vi "AUTON_Index.vi"(0 "Auton Array":dbl[][](array[numeric]), 5 "MeasuredHeading":dbl, 7 "LeftEncoder":dbl, 9 "RightEncoder":dbl) -> (4 "Right Drive":dbl, 6 "Left Drive":dbl, 8 "Harvester":dbl, 10 "Winch":dbl, 14 "Roller":dbl, 15 "Cam":dbl)   [LabVIEW 2013]
uses:
  Robot Global Data.vi
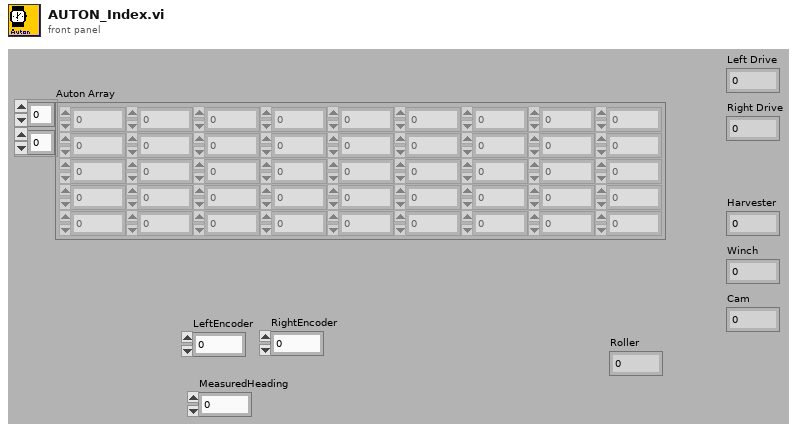
[diagram p1: front panel]
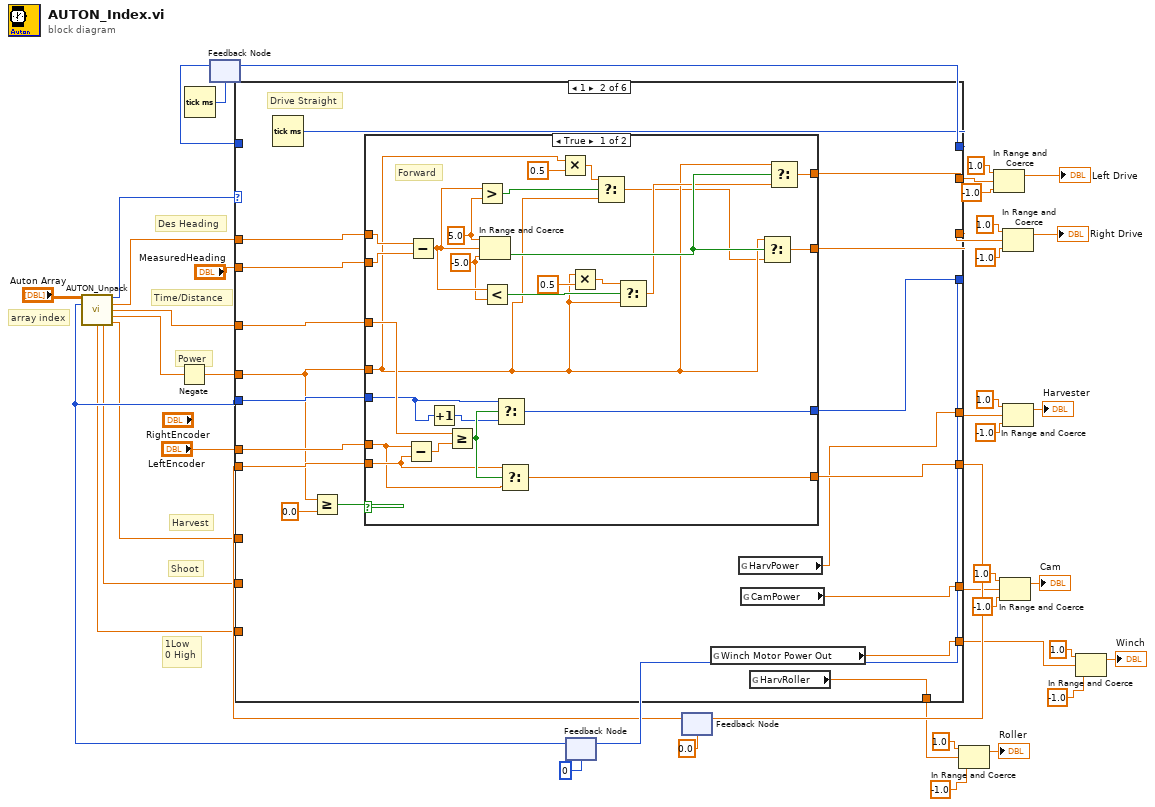
[diagram p0: block diagram]
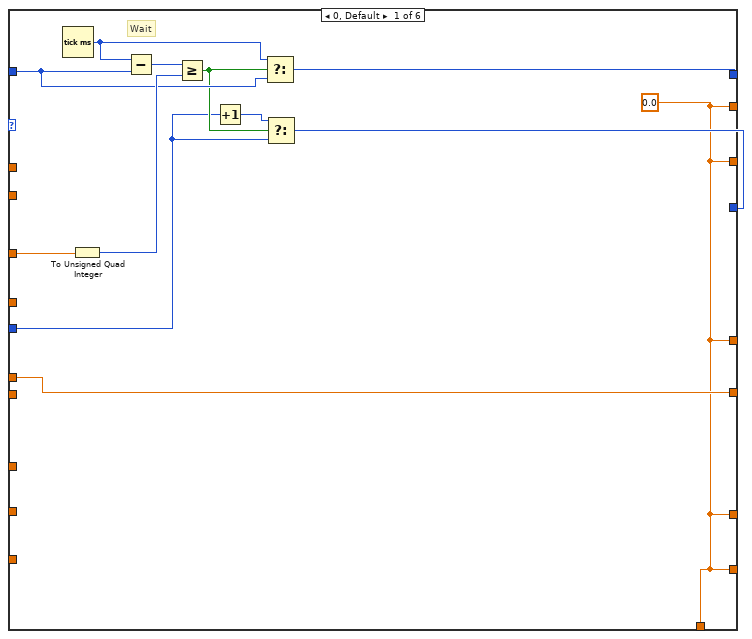
[diagram p2: hidden frame]
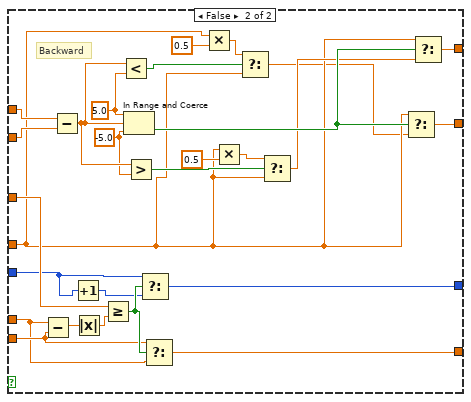
[diagram p3: hidden frame]
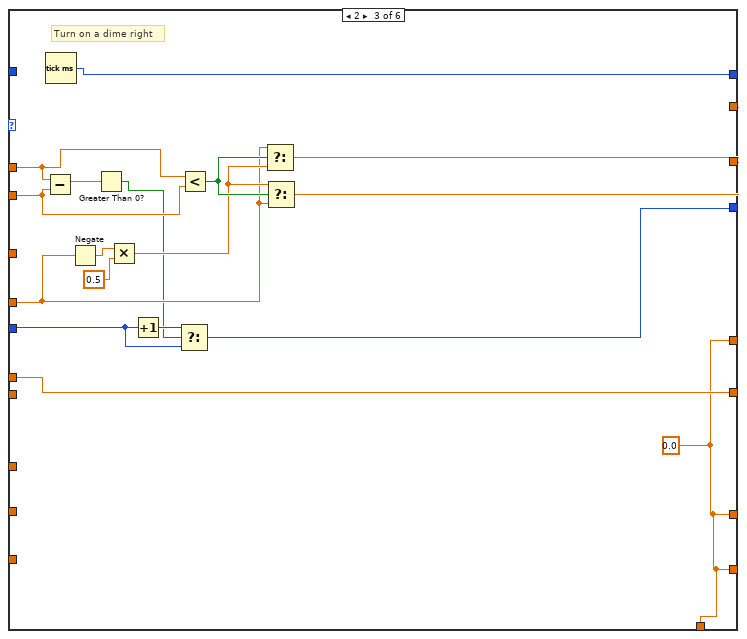
[diagram p4: hidden frame]
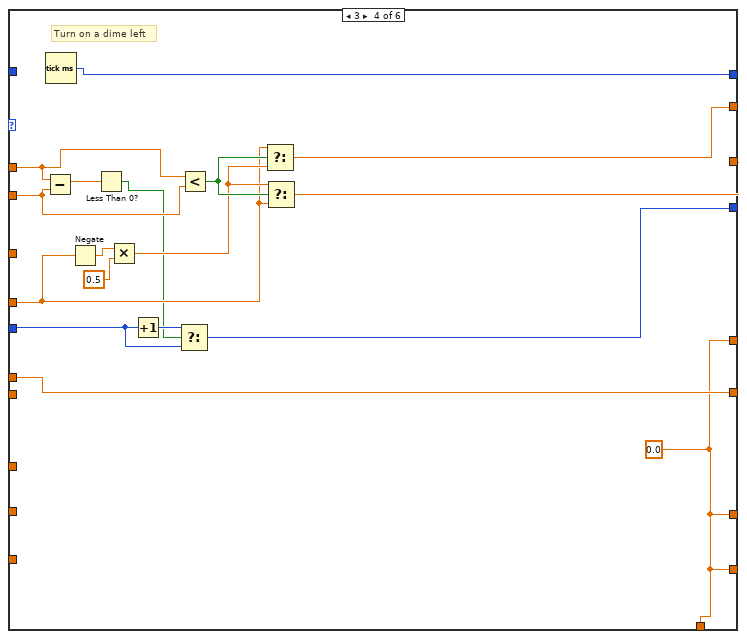
[diagram p5: hidden frame]
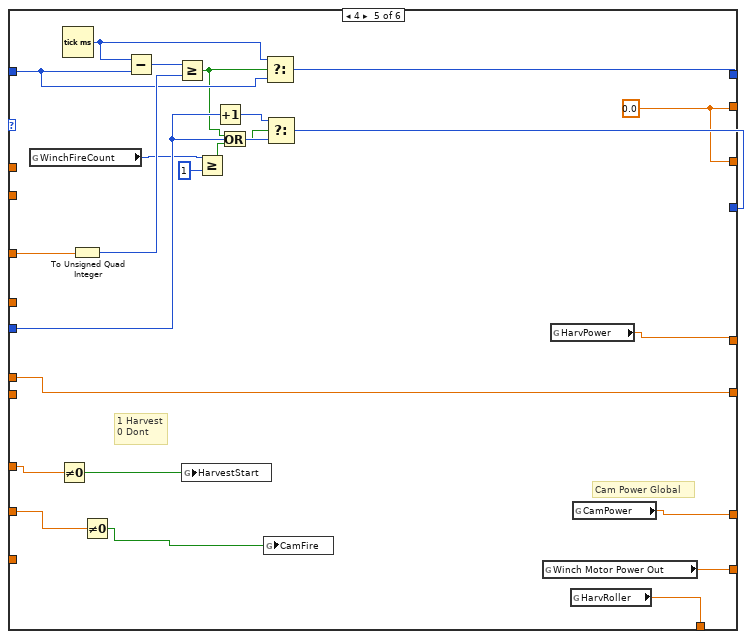
[diagram p6: hidden frame]
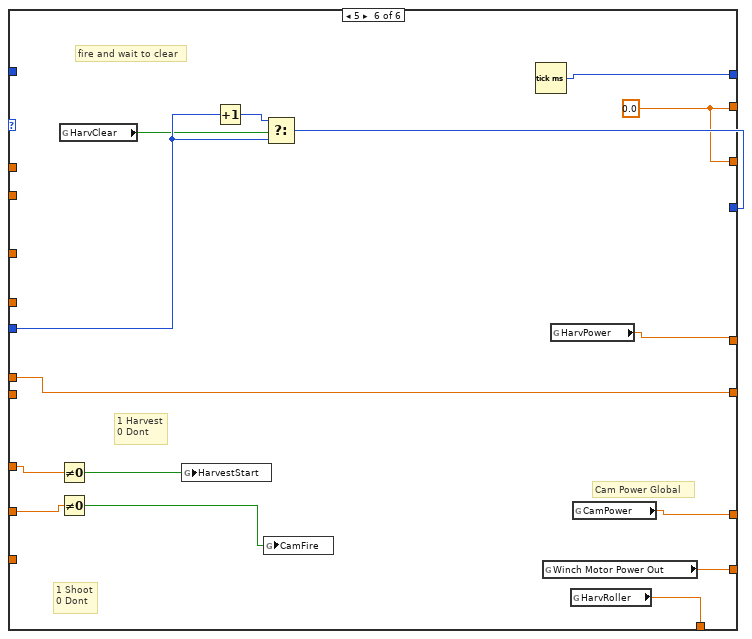
[diagram p7: hidden frame]
diagram:
  # "1Low\n0 High"
  # "Shoot"
  # "Harvest"
  # "Des Heading"
  # "Time/Distance"
  # "Power"
  # "array index"
  n1 = Tick Count (ms)() -> (millisecond timer value=w42:u32)
  n2 = feedback #1(w42) -> (w43:u32)
  n3 = feedback #2(0) -> (w23:i32)
  n4 = call "AUTON_Unpack.vi"("all rows"="Auton Array", "Index"=w23) -> ("Primitive ID"=w26:i16, "Desired Heading"=w25:dbl, "Time/Distance"=w24:dbl, "Power"=w11:dbl, "LowGear"=w1:dbl, "Shoot"=w8:dbl, "Harvest"=w9:dbl)  [unwired: 7 in]
  n5 = Negate(x=w11) -> (-x=w10:dbl)
  n6 = feedback #3(0.0) -> (w28:dbl)
  n7 = case shown="1" w26 {
    tunnel: [w48 w72 w139 w156 w178 w198] -> w30
    tunnel: w23 -> [w49 w67 w142 w159 w179 w199]
    tunnel: [w56 w64 w144 w161 w185 w189] -> w32
    tunnel: w43 -> [w53 _ _ _ w182 _]
    tunnel: w24 -> [w47 w73 _ _ w177 _]
    tunnel: w25 -> [_ w71 w137 w154 _ _]
    tunnel: [w45 w69 w140 w157 w176 w197] -> w40
    tunnel: [w45 w68 w141 w158 w176 w197] -> w33
    tunnel: w10 -> [_ w63 w131 w148 _ _]
    tunnel: "LeftEncoder" -> [w46 w65 w138 w155 w175 w196]
    tunnel: "MeasuredHeading" -> [_ w70 w136 w153 _ _]
    tunnel: w28 -> [_ w66 _ _ _ _]
    tunnel: [w46 w74 w138 w155 w175 w196] -> w27
    tunnel: [w45 w60 w128 w145 w173 w194] -> w13
    tunnel: [w45 w58 w128 w145 w174 w195] -> w12
    tunnel: w9 -> [_ _ _ _ w170 w192]
    tunnel: w8 -> [_ _ _ _ w172 w187]
    tunnel: [w45 w59 w128 w145 w171 w193] -> w7
    tunnel: [w45 w57 w128 w145 w167 w190] -> w3
    tunnel: w1 -> [_ _ _ _ _ _]
    frame 0, Default {
      w45 = 0.0 ("Numeric")
      # "Wait"
      n8 = Tick Count (ms)() -> (millisecond timer value=w52:u32)
      n9 = To Unsigned Quad Integer(1:w47) -> (0:w54:u64)
      n10 = Subtract(x=w52, y=w53) -> (x-y=w55:u32)
      n11 = Greater Or Equal?(x=w55, y=w54) -> (x >= y?=w51:bool)
      n12 = Increment(x=w49) -> (x+1=w50:i32)
      n13 = Select(t=w52, s=w51, f=w53) -> (s? t:f=w56:u32)
      n14 = Select(t=w50, s=w51, f=w49) -> (s? t:f=w48:i32)
    }
    frame 1 {
      # "Drive Straight"
      n15 = Tick Count (ms)() -> (millisecond timer value=w64:u32)
      n16 = Greater Or Equal?(x=w63, y=0.0) -> (x >= y?=w61:bool)
      n17 = case shown="True" w61 {
        tunnel: [w100 w127] -> w74
        tunnel: w73 -> [w98 w126]
        tunnel: [w96 w124] -> w72
        tunnel: w71 -> [w95 w123]
        tunnel: w70 -> [w94 w122]
        tunnel: [w92 w120] -> w69
        tunnel: [w91 w119] -> w68
        tunnel: w63 -> [w80 w108]
        tunnel: w67 -> [w77 w105]
        tunnel: w66 -> [w76 w104]
        tunnel: w65 -> [w75 w103]
        frame True {
          w88 = -5.0 ("lower limit")
          w90 = 5.0 ("upper limit")
          # "Forward"
          n18 = Subtract(x=w75, y=w76) -> (x-y=w99:dbl)
          n19 = Subtract(x=w95, y=w94) -> (x-y=w89:dbl)
          n20 = Increment(x=w77) -> (x+1=w78:i32)
          n21 = Greater Or Equal?(x=w98, y=w99) -> (x >= y?=w97:bool)
          n22 = Greater?(x=w89, y=w90) -> (0:w83:bool)
          n23 = In Range and Coerce(upper limit=w90, x=w89, lower limit=w88) -> (In Range?=w93:bool)  [unwired: 1 out]
          n24 = Less?(x=w89, y=w88) -> (x < y?=w87:bool)
          n25 = Select(t=w77, s=w97, f=w78) -> (s? t:f=w96:i32)
          n26 = Select(t=w76, s=w97, f=w75) -> (s? t:f=w100:dbl)
          n27 = Multiply(x=w80, y=0.5) -> (x*y=w82:dbl)
          n28 = Multiply(x=w80, y=0.5) -> (x*y=w85:dbl)
          n29 = Select(t=w82, s=w83, f=w80) -> (s? t:f=w79:dbl)
          n30 = Select(t=w85, s=w87, f=w80) -> (s? t:f=w84:dbl)
          n31 = Select(t=w80, s=w93, f=w79) -> (s? t:f=w91:dbl)
          n32 = Select(t=w80, s=w93, f=w84) -> (s? t:f=w92:dbl)
        }
        frame False {
          w116 = -5.0 ("lower limit")
          w118 = 5.0 ("upper limit")
          # "Backward"
          n33 = Subtract(x=w103, y=w104) -> (x-y=w101:dbl)
          n34 = Subtract(x=w123, y=w122) -> (x-y=w117:dbl)
          n35 = Increment(x=w105) -> (x+1=w106:i32)
          n36 = Absolute Value(x=w101) -> (abs(x)=w102:dbl)
          n37 = Greater Or Equal?(x=w126, y=w102) -> (x >= y?=w125:bool)
          n38 = Less?(x=w117, y=w118) -> (x < y?=w111:bool)
          n39 = In Range and Coerce(upper limit=w118, x=w117, lower limit=w116) -> (In Range?=w121:bool)  [unwired: 1 out]
          n40 = Greater?(x=w117, y=w116) -> (0:w115:bool)
          n41 = Select(t=w105, s=w125, f=w106) -> (s? t:f=w124:i32)
          n42 = Select(t=w104, s=w125, f=w103) -> (s? t:f=w127:dbl)
          n43 = Multiply(x=w108, y=0.5) -> (x*y=w110:dbl)
          n44 = Multiply(x=w108, y=0.5) -> (x*y=w113:dbl)
          n45 = Select(t=w110, s=w111, f=w108) -> (s? t:f=w107:dbl)
          n46 = Select(t=w113, s=w115, f=w108) -> (s? t:f=w112:dbl)
          n47 = Select(t=w108, s=w121, f=w107) -> (s? t:f=w119:dbl)
          n48 = Select(t=w108, s=w121, f=w112) -> (s? t:f=w120:dbl)
        }
      }
      n49 = global read "Robot Global Data.vi" "Winch Motor Power Out"() -> (w59:dbl)
      n50 = global read "Robot Global Data.vi" "HarvPower"() -> (w58:dbl)
      n51 = global read "Robot Global Data.vi" "CamPower"() -> (w60:dbl)
      n52 = global read "Robot Global Data.vi" "HarvRoller"() -> (w57:dbl)
    }
    frame 2 {
      w128 = 0.0 ("Numeric")
      # "Turn on a dime right"
      n53 = Subtract(x=w137, y=w136) -> (x-y=w130:dbl)
      n54 = Tick Count (ms)() -> (millisecond timer value=w144:u32)
      n55 = Negate(x=w131) -> (-x=w134:dbl)
      n56 = Greater Than 0?(x=w130) -> (x > 0?=w129:bool)
      n57 = Multiply(x=w134, y=0.5) -> (x*y=w132:dbl)
      n58 = Increment(x=w142) -> (x+1=w143:i32)
      n59 = Select(t=w143, s=w129, f=w142) -> (s? t:f=w139:i32)
      n60 = Less?(x=w137, y=w136) -> (x < y?=w135:bool)
      n61 = Select(t=w131, s=w135, f=w132) -> (s? t:f=w140:dbl)
      n62 = Select(t=w132, s=w135, f=w131) -> (s? t:f=w141:dbl)
    }
    frame 3 {
      w145 = 0.0 ("Numeric")
      # "Turn on a dime left"
      n63 = Subtract(x=w154, y=w153) -> (x-y=w147:dbl)
      n64 = Tick Count (ms)() -> (millisecond timer value=w161:u32)
      n65 = Negate(x=w148) -> (-x=w151:dbl)
      n66 = Less Than 0?(x=w147) -> (x < 0?=w146:bool)
      n67 = Multiply(x=w151, y=0.5) -> (x*y=w149:dbl)
      n68 = Increment(x=w159) -> (x+1=w160:i32)
      n69 = Select(t=w160, s=w146, f=w159) -> (s? t:f=w156:i32)
      n70 = Less?(x=w154, y=w153) -> (x < y?=w152:bool)
      n71 = Select(t=w148, s=w152, f=w149) -> (s? t:f=w157:dbl)
      n72 = Select(t=w149, s=w152, f=w148) -> (s? t:f=w158:dbl)
    }
    frame 4 {
      w176 = 0.0 ("Numeric")
      # "1 Harvest\n0 Dont"
      # "Cam Power Global"
      n73 = global read "Robot Global Data.vi" "WinchFireCount"() -> (w163:i32)
      n74 = Not Equal To 0?(x=w170) -> (x != 0?=w169:bool)
      n75 = Tick Count (ms)() -> (millisecond timer value=w181:u32)
      n76 = To Unsigned Quad Integer(1:w177) -> (0:w183:u64)
      n77 = Not Equal To 0?(x=w172) -> (x != 0?=w168:bool)
      n78 = Subtract(x=w181, y=w182) -> (x-y=w184:u32)
      n79 = Greater Or Equal?(x=w184, y=w183) -> (x >= y?=w165:bool)
      n80 = global write "Robot Global Data.vi" "HarvestStart"(w169) -> ()
      n81 = Greater Or Equal?(x=w163, y=1) -> (x >= y?=w164:bool)
      n82 = Increment(x=w179) -> (x+1=w180:i32)
      n83 = Or(x=w165, y=w164) -> (x .or. y?=w166:bool)
      n84 = global write "Robot Global Data.vi" "CamFire"(w168) -> ()
      n85 = Select(t=w181, s=w165, f=w182) -> (s? t:f=w185:u32)
      n86 = Select(t=w180, s=w166, f=w179) -> (s? t:f=w178:i32)
      n87 = global read "Robot Global Data.vi" "Winch Motor Power Out"() -> (w171:dbl)
      n88 = global read "Robot Global Data.vi" "HarvPower"() -> (w174:dbl)
      n89 = global read "Robot Global Data.vi" "HarvRoller"() -> (w167:dbl)
      n90 = global read "Robot Global Data.vi" "CamPower"() -> (w173:dbl)
    }
    frame 5 {
      w197 = 0.0 ("Numeric")
      # "fire and wait to clear"
      # "1 Harvest\n0 Dont"
      # "1 Shoot\n0 Dont"
      # "Cam Power Global"
      n91 = Not Equal To 0?(x=w192) -> (x != 0?=w191:bool)
      n92 = Not Equal To 0?(x=w187) -> (x != 0?=w186:bool)
      n93 = global read "Robot Global Data.vi" "HarvClear"() -> (w188:bool)
      n94 = global write "Robot Global Data.vi" "HarvestStart"(w191) -> ()
      n95 = Increment(x=w199) -> (x+1=w200:i32)
      n96 = global write "Robot Global Data.vi" "CamFire"(w186) -> ()
      n97 = Select(t=w200, s=w188, f=w199) -> (s? t:f=w198:i32)
      n98 = Tick Count (ms)() -> (millisecond timer value=w189:u32)
      n99 = global read "Robot Global Data.vi" "Winch Motor Power Out"() -> (w193:dbl)
      n100 = global read "Robot Global Data.vi" "HarvPower"() -> (w195:dbl)
      n101 = global read "Robot Global Data.vi" "HarvRoller"() -> (w190:dbl)
      n102 = global read "Robot Global Data.vi" "CamPower"() -> (w194:dbl)
    }
  }
  n103 = feedback-in #1(w32) -> ()
  n104 = feedback-in #2(w30) -> ()
  n105 = feedback-in #3(w27) -> ()
  n106 = In Range and Coerce(upper limit=1.0, x=w3, lower limit=-1.0) -> (coerced(x)=→"Roller":dbl)  [unwired: 1 out]
  n107 = In Range and Coerce(upper limit=1.0, x=w40, lower limit=-1.0) -> (coerced(x)=→"Left Drive":dbl)  [unwired: 1 out]
  n108 = In Range and Coerce(upper limit=1.0, x=w13, lower limit=-1.0) -> (coerced(x)=→"Cam":dbl)  [unwired: 1 out]
  n109 = In Range and Coerce(upper limit=1.0, x=w33, lower limit=-1.0) -> (coerced(x)=→"Right Drive":dbl)  [unwired: 1 out]
  n110 = In Range and Coerce(upper limit=1.0, x=w12, lower limit=-1.0) -> (coerced(x)=→"Harvester":dbl)  [unwired: 1 out]
  n111 = In Range and Coerce(upper limit=1.0, x=w7, lower limit=-1.0) -> (coerced(x)=→"Winch":dbl)  [unwired: 1 out]
